vi "-Build_Connect_Error.vi"(8 "error in (no error)":errorcluster, 11 "Postgres Connector In":refnum<class "Postgres Connector.lvclass">) -> (0 "error out":errorcluster)   [LabVIEW 2019, in "PG_LIB.lvlib" / "Postgres Connector.lvclass"]
doc: "This VI return an error if the connection with the database could not be establish"
uses:
  Postgres Connector.lvclass
  Postgres Connector.lvclass/Postgres Connector.ctl
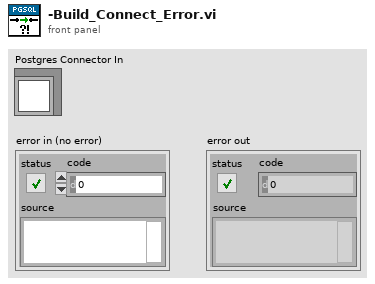
[diagram p1: front panel]
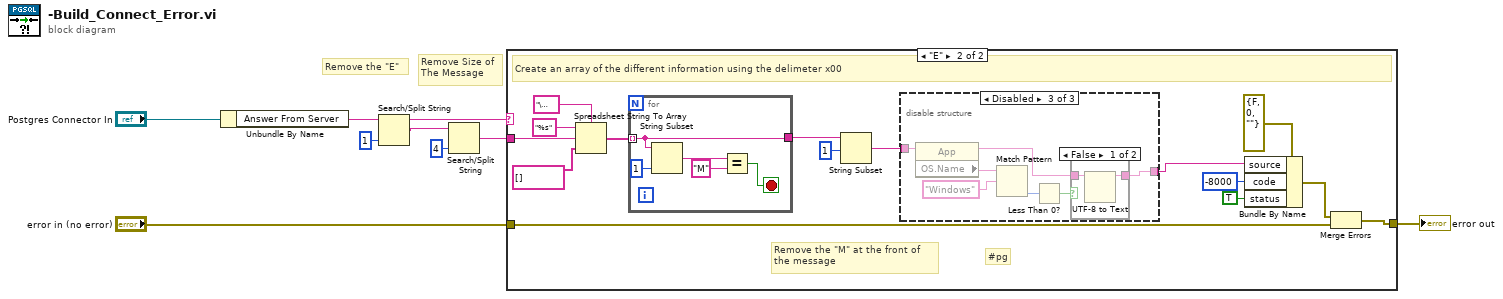
[diagram p0: block diagram]
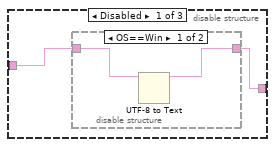
[diagram p3: hidden frame]
diagram:
  # "Remove Size of\nThe Message"
  # "Remove the \"E\""
  n1 = Unbundle By Name("Postgres Connector In") -> ("Answer From Server"=w4:string)
  n2 = Search/Split String(string=w4, offset (0)=1 ("length (rest)")) -> (substring before match=w5:string, match + rest of string=w2:string)  [unwired: 1 in, 1 out]
  n3 = Search/Split String(string=w2, offset (0)=4 ("length (rest)")) -> (match + rest of string=w1:string)  [unwired: 1 in, 2 out]
  n4 = case shown="\"E\"" w5 {
    tunnel: "error in (no error)" -> [w10 w21]
    tunnel: [w10 w23] -> w7
    tunnel: w1 -> [_ w16]
    frame "False", Default {
    }
    frame "E" {
      # "#pg"
      # "Remove the \"M\" at the front of\nthe message"
      # "Create an array of the different information using the delimeter x00"
      n5 = Spreadsheet String To Array(delimiter (Tab)="\u0000", format string="%s", spreadsheet string=w16, array type (2D Dbl)=string[] []) -> (array=w14:string[])
      n6 = for {
        tunnel: w14 -> [w43] mode=indexing
        tunnel: [w43] -> w13
        stop <- w41 stop-if-true
        n7 = String Subset(string=w43, length (rest)=1 ("length (rest)")) -> (substring=w44:string)  [unwired: 1 in]
        n8 = Equal?(x=w44, y="M") -> (x = y?=w41:bool)
      }
      n9 = String Subset(string=w13, offset (0)=1) -> (substring=w12:string)  [unwired: 1 in]
      n10 = disable-structure shown="Disabled" {
        disable-tunnel: [w27 w31 w32] -> w11
        disable-tunnel: w12 -> [w26 w31 w33]
        frame Disabled {
          n11 = disable-structure shown="OS==Win" {
            disable-tunnel: [w29 w30] -> w27
            disable-tunnel: w26 -> [w28 w30]
            frame condition #0 {
              n12 = UTF-8 to Text(11:w28) -> (3:w29:string)  [unwired: 2 in, 1 out]
            }
            frame condition #1 (active) {
            }
          }
        }
        frame Enabled {
        }
        frame Disabled {
          n13 = property class="App"() -> ("OS.Name"=w35:string)  [unwired: 2 in, 2 out]
          n14 = Match Pattern(string=w35, regular expression="Windows") -> (offset past match=w36:i32)  [unwired: 1 in, 3 out]
          n15 = Less Than 0?(x=w36) -> (x < 0?=w37:bool)
          n16 = case shown="False" w37 {
            tunnel: [w39 w40] -> w32
            tunnel: w33 -> [w38 w40]
            frame False {
              n17 = UTF-8 to Text(11:w38) -> (3:w39:string)  [unwired: 2 in, 1 out]
            }
            frame True {
            }
          }
        }
      }
      n18 = Bundle By Name(cluster=errorcluster {"status"=FALSE, "code"=0, "source"=""} ("error in (no error)"), "source"=w11, "code"=-8000, "status"=TRUE) -> (w22:errorcluster)
      n19 = Merge Errors(w22, w21) -> (w23:errorcluster)
    }
  }
  "error out" <- w7
